vi "MARS_MagnetometerHMC588L_I2C_Get.vi"(8 "error in":errorcluster, 11 "I2CDevRef":T2={"DevStatus"={"status"=FALSE, "code"=0, "source"=""}, "Controller"=enum."Controller 1", "Device Address"=0, "Handle"=0, "I2C Bus"=enum."Invalid"} {"Device Address" format="%.0x"}) -> (0 "error out":errorcluster, 2 "Magnetometer Reading":T1, 3 "I2CDevRef 2":T2={"DevStatus"={"status"=FALSE, "code"=0, "source"=""}, "Controller"=enum."Controller 1", "Device Address"=0, "Handle"=0, "I2C Bus"=enum."Invalid"} {"Device Address" format="%.0x"})   [LabVIEW 2014]
uses:
  <vilib>/Rock Robotics/WPI/I2C/WPI_I2CDevRef.ctl
  <vilib>/Rock Robotics/SystemInterfaces/Typedef/FPGA_TypedefDigitalModule.ctl
  <vilib>/Rock Robotics/SystemInterfaces/i2clib/i2c_bus.ctl
  Magnetometer Readings Cluster.ctl
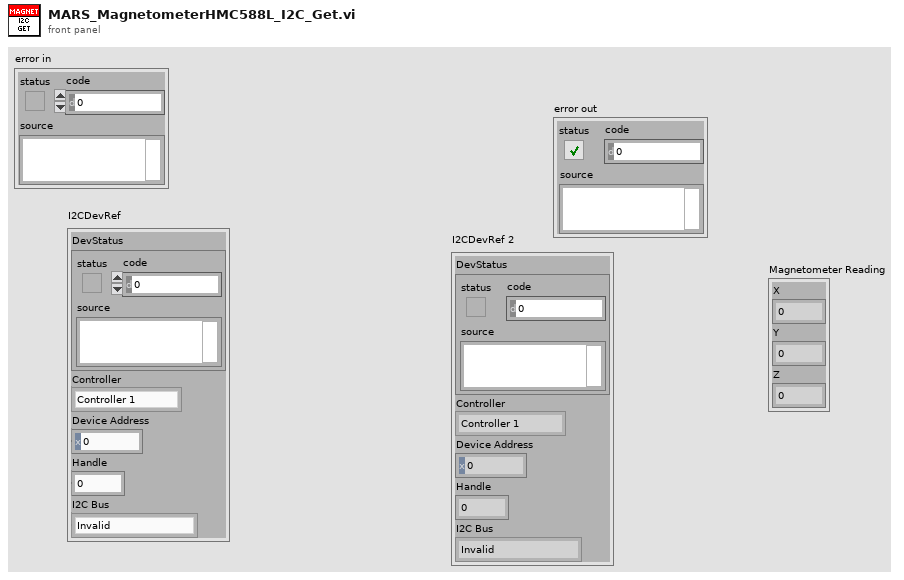
[diagram p1: front panel]
types:
  T1 = typedef "Magnetometer Readings Cluster.ctl" = cluster{"X":i32, "Y":i32, "Z":i32}
  T2 = typedef "WPI_I2CDevRef.ctl" = cluster{"DevStatus":errorcluster, "Controller":T3, "Device Address":u8, "Handle":i32, "I2C Bus":T4}
  T3 = typedef "FPGA_TypedefDigitalModule.ctl" = enum16{"Controller 1"}
  T4 = typedef "i2c_bus.ctl" = enum16{"I2C On-Board", "I2C MXP", "Invalid"}
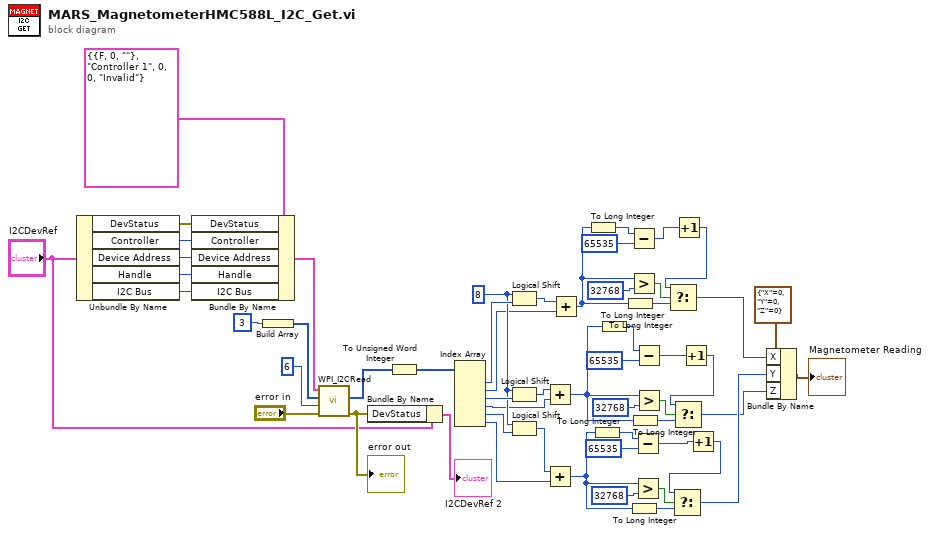
[diagram p0: block diagram]
diagram:
  w39 = u8 8 ("x")
  n1 = Unbundle By Name("I2CDevRef") -> ("DevStatus"=w51:errorcluster, "Controller"=w50:T3, "Device Address"=w49:u8, "Handle"=w48:i32, "I2C Bus"=w47:T4)
  n2 = Bundle By Name(cluster=T2 {"DevStatus"={"status"=FALSE, "code"=0, "source"=""}, "Controller"=enum."Controller 1", "Device Address"=0, "Handle"=0, "I2C Bus"=enum."Invalid"} ("input cluster"), "DevStatus"=w51, "Controller"=w50, "Device Address"=w49, "Handle"=w48, "I2C Bus"=w47) -> (w43:T2)
  n3 = Build Array(u8 3 ("Data To Send")) -> (w44:u8[])
  n4 = call <vilib>:"WPI_I2CRead.vi"("error in (no error)"="error in", "I2CBytesToRead"=u8 6, "I2CRegister"=w44, "I2CDevRef"=w43) -> ("error out"=w53:errorcluster, "Data Out"=w36:u8[])  [unwired: 6 out]
  "error out" <- w53
  n5 = Bundle By Name(cluster="I2CDevRef", "DevStatus"=w53) -> (→"I2CDevRef 2":T2)
  n6 = To Unsigned Word Integer(number=w36) -> (unsigned 16bit integer=w37:u16[])
  n7 = Index Array(array=w37) -> (element #1=w41:u16, element #2=w34:u16, element #3=w40:u16, element #4=w32:u16, element #5=w38:u16, element #6=w30:u16)  [unwired: 6 in]
  n8 = Logical Shift(y=w39, x=w41) -> (x << y=w35:u16)
  n9 = Logical Shift(y=w39, x=w40) -> (x << y=w33:u16)
  n10 = Logical Shift(y=w39, x=w38) -> (x << y=w31:u16)
  n11 = Add(x=w33, y=w32) -> (x+y=w18:u16)
  n12 = Add(x=w31, y=w30) -> (x+y=w12:u16)
  n13 = Add(x=w35, y=w34) -> (x+y=w25:u16)
  n14 = To Long Integer(number=w25) -> (32bit integer=w27:i32)
  n15 = To Long Integer(number=w12) -> (32bit integer=w15:i32)
  n16 = To Long Integer(number=w18) -> (32bit integer=w21:i32)
  n17 = To Long Integer(number=w25) -> (32bit integer=w24:i32)
  n18 = Subtract(x=w27, y=65535) -> (x-y=w11:i32)
  n19 = Greater?(x=w25, y=u16 32768) -> (0:w29:bool)
  n20 = To Long Integer(number=w12) -> (32bit integer=w13:i32)
  n21 = To Long Integer(number=w18) -> (32bit integer=w19:i32)
  n22 = Subtract(x=w15, y=65535) -> (x-y=w7:i32)
  n23 = Greater?(x=w12, y=u16 32768) -> (0:w17:bool)
  n24 = Subtract(x=w21, y=65535) -> (x-y=w9:i32)
  n25 = Greater?(x=w18, y=u16 32768) -> (0:w23:bool)
  n26 = Increment(x=w11) -> (x+1=w10:i32)
  n27 = Select(t=w10, s=w29, f=w24) -> (s? t:f=w4:i32)
  n28 = Increment(x=w9) -> (x+1=w8:i32)
  n29 = Select(t=w8, s=w23, f=w19) -> (s? t:f=w2:i32)
  n30 = Increment(x=w7) -> (x+1=w6:i32)
  n31 = Select(t=w6, s=w17, f=w13) -> (s? t:f=w3:i32)
  n32 = Bundle By Name(cluster=T1 {"X"=0, "Y"=0, "Z"=0}, "X"=w4, "Y"=w3, "Z"=w2) -> (→"Magnetometer Reading":T1)
